vi "SHCWV Specific Heat Capacity of Water Vapor (J to Kg K).vi"(1 "Tceg":dbl[unit]) -> (0 "SHCWV":dbl[unit])   [LabVIEW 2018]
panel:
  out "SHCWV\nSpecific Heat Capacity of Water Vapor\nSHCWV=1.8234+(0.00031229*Tk)":dbl[unit](knob)
  out "Temprature Of Input Air\nKelvin Degree":dbl[unit](slide) scale=273.0..373.0
  out "Tk":dbl[unit]
  out "Temprature Of Input Air\nCentigrade Degree":dbl[unit](slide) scale=0.0..100.0
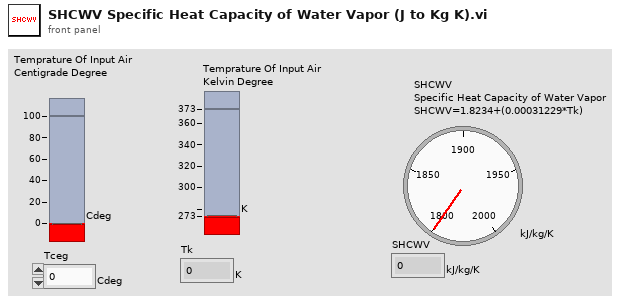
[diagram p1: front panel]
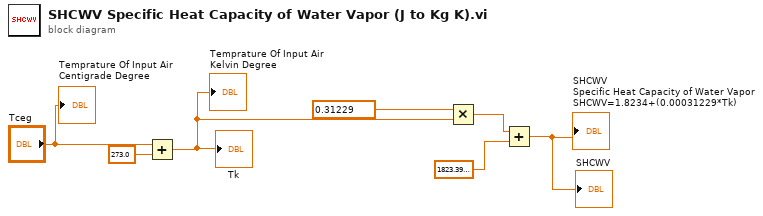
[diagram p0: block diagram]
diagram:
  n1 = Add(x="Tceg", y=dbl[unit] 273.0) -> (x+y=w3:dbl[unit])
  "Tk" <- w3
  "Temprature Of Input Air\nKelvin Degree" <- w3
  n2 = Multiply(x=dbl[unit] 0.31229, y=w3) -> (x*y=w5:dbl[unit])
  n3 = Add(x=w5, y=dbl[unit] 1823.3999999999999) -> (x+y=→"SHCWV\nSpecific Heat Capacity of Water Vapor\nSHCWV=1.8234+(0.00031229*Tk)" →"SHCWV":dbl[unit])
  "Temprature Of Input Air\nCentigrade Degree" <- "Tceg"
